vi "2D to YX.vi"(8 "error in (no error)":errorcluster, 10 "Y Array":dbl[](array[numeric]), 11 "2D Z Array":dbl[][](array[numeric])) -> (0 "error out":errorcluster, 3 "XY-data out":cluster{"X-array":dbl[], "Y-array":dbl[]}[](array[cluster]) {"Y-array" format="%.2p"; "X-array" format="%.2p"})   [LabVIEW 2019, in "xy_utilities.lvlib"]
doc: "Convert <b>2D Z Array</b> and <b>Y Array</b> to Array of <b>XY-Data</b> (where <b>XY = YZ</b>)"
uses:
  xy_utilities.lvlib
panel:
  out "Numeric":i32
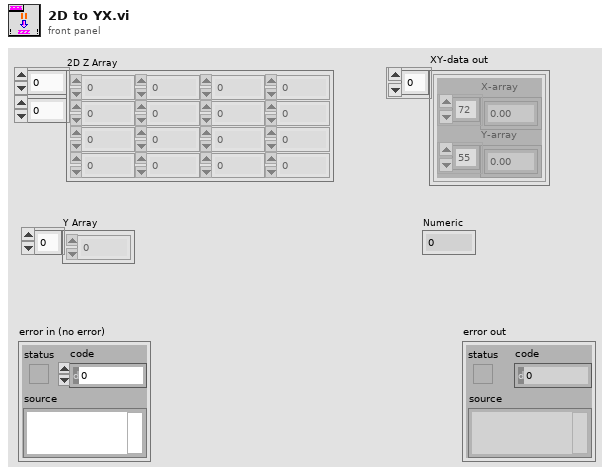
[diagram p1: front panel]
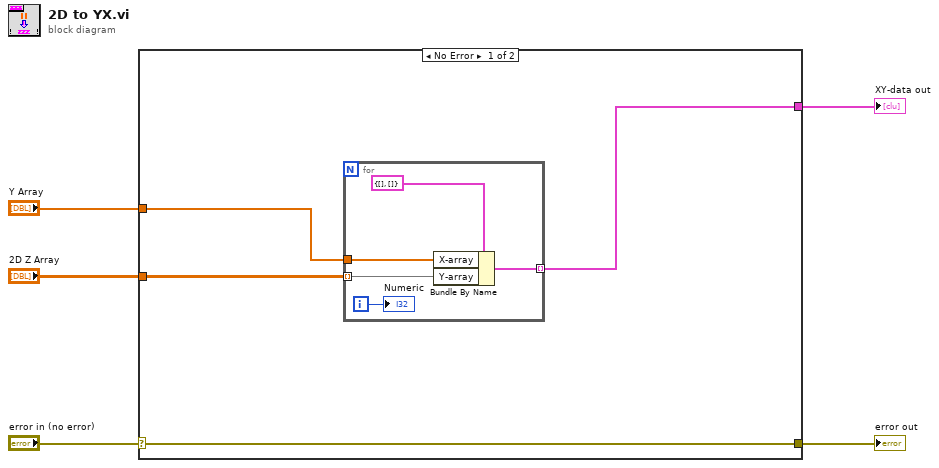
[diagram p0: block diagram]
diagram:
  n1 = case shown="No Error" "error in (no error)" {
    selector: "error in (no error)" -> [w9 w15]
    tunnel: [w9 w15] -> w4
    tunnel: [w7 _] -> w3
    tunnel: "2D Z Array" -> [w6 _]
    tunnel: "Y Array" -> [w8 _]
    frame No Error {
      n2 = for {
        tunnel: w6 -> [w13] mode=indexing
        tunnel: w8 -> [w11]
        tunnel: [w12] -> w7 mode=indexing
        i -> [w10]
        n3 = Bundle By Name(cluster=cluster{"X-array":dbl[], "Y-array":dbl[]} {"X-array"=[], "Y-array"=[]}, "X-array"=w11, "Y-array"=w13) -> (w12:cluster{"X-array":dbl[], "Y-array":dbl[]})
        "Numeric" <- w10
      }
    }
    frame Error {
    }
  }
  "error out" <- w4
  "XY-data out" <- w3
